vi "New Styled Paragraph.vi"(7 "xwpfParagraph Type":refnum<class "xwpfParagraph.lvclass">, 8 "error in (no error)":errorcluster, 9 "Type":T1(ring), 10 "Paragraph.Text":string, 11 "Paragraph.Ref":refnum<k24>) -> (0 "error out":errorcluster, 3 "xwpfParagraph out":refnum<class "xwpfParagraph.lvclass">)   [LabVIEW 2017, in "Word_Specific.lvlib" / "xwpfParagraph.lvclass"]
uses:
  xwpfParagraph.lvclass
  C:/Users/Neo/Desktop/Dev_Tools_BR/LabVIEW_NPOI/lib/NPOI 2.1.1/NPOI.OOXML.dll
  lib/NPOI 2.1.1/NPOI.OOXML.dll
  xwpfParagraph.lvclass/xwpfParagraph.ctl
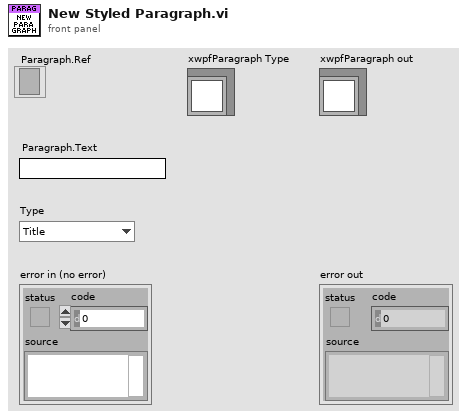
[diagram p1: front panel]
types:
  T1 = enum16{"Title", "Heading 1", "Heading 2", "Heading 3", "Normal", "Figure", "Page Break"}
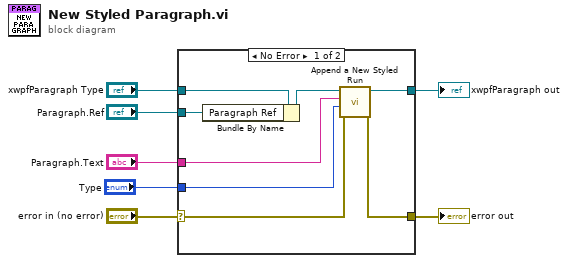
[diagram p0: block diagram]
diagram:
  n1 = case shown="No Error" "error in (no error)" {
    selector: "error in (no error)" -> [w12 w17]
    tunnel: [w14 w17] -> w6
    tunnel: [w15 w16] -> w4
    tunnel: "xwpfParagraph Type" -> [w11 w16]
    tunnel: "Paragraph.Ref" -> [w9 _]
    tunnel: "Paragraph.Text" -> [w13 _]
    tunnel: "Type" -> [w8 _]
    frame No Error {
      n2 = Bundle By Name(cluster=w11, "Paragraph Ref"=w9) -> (w10:refnum<class "xwpfParagraph.lvclass">)
      n3 = call "Append a New Styled Run.vi"("error in (no error)"=w12, "Run Type"=w8, "Text"=w13, "xwpfParagraph in"=w10) -> ("error out"=w14:errorcluster, "xwpfParagraph out"=w15:refnum<class "xwpfParagraph.lvclass">)  [unwired: 6 in]
    }
    frame Error {
    }
  }
  "error out" <- w6
  "xwpfParagraph out" <- w4
